vi "Elevator.vi"() -> ()   [LabVIEW 2020]
doc: "Main Vi for the Elevator project that will launch the application and all its submodules"
uses:
  Controller/Controls/Application Event Message.ctl
  Controller/Controls/Application Modules.ctl
  Controller/Controls/Application Events.ctl
  Error Module/Controls/Module Message.ctl
  Configuration Database/Controls/FGV Mode.ctl
  Controller/Controller.lvlib
  Error Module/Error Handler.lvlib
  Configuration Database/Configuration Database.lvlib
  Sensor Interface/Sensor Interface.lvlib
  User Console/User Console.lvlib
  Display Console/Display Console.lvlib
panel:
  in  "Simulate Configuration Database?":bool
  in  "Simulate Sensor Interface?":bool
  in  "Simulate Display Console?":bool
  in  "Simulate User Console?":bool
  out "error out":errorcluster
  in  "error in":errorcluster
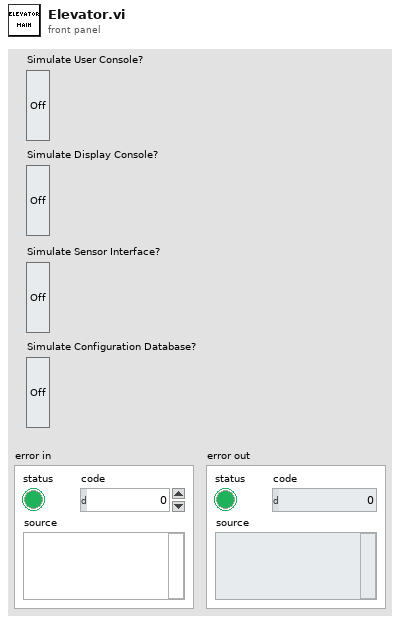
[diagram p1: front panel]
types:
  T1 = typedef "Configuration Database.lvlib/FGV Mode.ctl" = enum16{"Initialize", "Get", "Update", "Close"}
  T2 = typedef "Error Handler.lvlib/Module Message.ctl" = cluster{"Source":T3, "Error":errorcluster}
  T3 = typedef "Controller.lvlib/Application Modules.ctl" = enum16{"Controller", "User Console", "Display Console", "Sensor Interface", "Configuration Database", "Error Module"}
  T4 = typedef "Controller.lvlib/Application Event Message.ctl" = cluster{"Source":T3, "Event":T5, "Data":variant}
  T5 = typedef "Controller.lvlib/Application Events.ctl" = enum16{"Controller: Initialize", "Controller: Initialize Start And Move State", "Controller: Initialize Analysis State", "Controller: Initialize Continue Travel State", "Controller: Initialize Stop At Floor", "Controller: Initialize Open And Close Door Sequence", "Controller: Initialize No Request Remaining", "Controller: Initialize Emergency Call", "Controller: Initialize Terminate Process", "Controller: Publish State", "UI: Elevator Call", "UI: Broadcast State", "UI: Next Destination Reached", "UI: Timeout Reached", "UI: Emergency Call", "UI: Terminate State", "UI: Door Opened", "UI: Door Closed", "UI: Floor Reached", "UI: Door About To Close"}
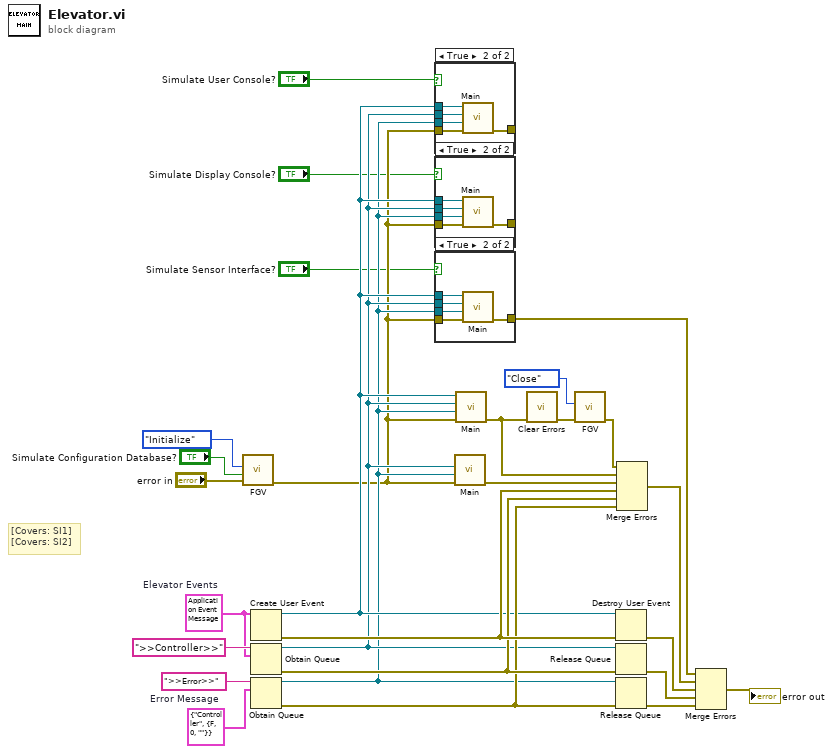
[diagram p0: block diagram]
diagram:
  w21 = T2 {"Source"=enum."Controller", "Error"={"status"=FALSE, "code"=0, "source"=""}}  # Error Message
  w22 = T4 {"Source"=enum."Controller", "Event"=enum."Controller: Initialize", "Data"=variant}  # Elevator Events
  # "[Covers: SI1] \n[Covers: SI2]"
  n1 = call "FGV.vi"("error in"="error in", "Use Simulated?"="Simulate Configuration Database?", "Mode"=FGV_Mode."Initialize") -> ("error out"=w8:errorcluster)  [unwired: 7 in, 1 out]
  n2 = Create User Event(user event datatype=w22) -> (user event=w11:refnum<user-event>, error out=w16:errorcluster)  [unwired: 1 in]
  n3 = Obtain Queue(name (unnamed)=">>Controller>>", element data type=w22) -> (queue out=w10:refnum<queue>, error out=w15:errorcluster)  [unwired: 3 in, 1 out]
  n4 = Obtain Queue(name (unnamed)=">>Error>>", element data type=w21) -> (queue out=w9:refnum<queue>, error out=w14:errorcluster)  [unwired: 3 in, 1 out]
  n5 = case shown="True" "Simulate User Console?" {
    tunnel: w8 -> [w29 w34]
    tunnel: w9 -> [_ w33]
    tunnel: w10 -> [_ w32]
    tunnel: w11 -> [_ w31]
    tunnel: [w29 w30] -> _
    frame False {
    }
    frame True {
      n6 = call "Main.vi"("error in"=w34, "Error Queue"=w33, "Controller Queue"=w32, "Application Events"=w31) -> ("error out"=w30:errorcluster)  [unwired: 7 in]
    }
  }
  n7 = case shown="True" "Simulate Display Console?" {
    tunnel: w8 -> [w35 w40]
    tunnel: w9 -> [_ w39]
    tunnel: w10 -> [_ w38]
    tunnel: w11 -> [_ w37]
    tunnel: [w35 w36] -> _
    frame False {
    }
    frame True {
      n8 = call "Main.vi"("error in"=w40, "Error Queue"=w39, "Controller Queue"=w38, "Application Events"=w37) -> ("error out"=w36:errorcluster)  [unwired: 7 in]
    }
  }
  n9 = case shown="True" "Simulate Sensor Interface?" {
    tunnel: w8 -> [w41 w46]
    tunnel: w9 -> [_ w45]
    tunnel: w10 -> [_ w44]
    tunnel: w11 -> [_ w43]
    tunnel: [w41 w42] -> w12
    frame False {
    }
    frame True {
      n10 = call "Main.vi"("error in"=w46, "Error Queue"=w45, "Controller Queue"=w44, "Application Events"=w43) -> ("error out"=w42:errorcluster)  [unwired: 7 in]
    }
  }
  n11 = call "Main.vi"("error in"=w8, "Error Queue"=w9, "Controller Queue"=w10) -> ("error out"=w17:errorcluster)  [unwired: 8 in]
  n12 = call "Main.vi"("error in"=w8, "Error Queue"=w9, "Controller Queue"=w10, "Application Events"=w11) -> ("error out"=w3:errorcluster)  [unwired: 7 in]
  n13 = call <vilib>:"Clear Errors.vi"("error in (no error)"=w3) -> ("error out"=w2:errorcluster)  [unwired: 5 in, 1 out]
  n14 = call "FGV.vi"("error in"=w2, "Mode"=FGV_Mode."Close") -> ("error out"=w4:errorcluster)  [unwired: 8 in, 1 out]
  n15 = Destroy User Event(user event=w11, error in=w16) -> (error out=w28:errorcluster)
  n16 = Release Queue(queue=w10, error in (no error)=w15) -> (error out=w27:errorcluster)  [unwired: 1 in, 2 out]
  n17 = Release Queue(queue=w9, error in (no error)=w14) -> (error out=w26:errorcluster)  [unwired: 1 in, 2 out]
  n18 = Merge Errors(w4, w3, w17, w16, w15, w14) -> (w13:errorcluster)
  n19 = Merge Errors(w12, w13, w28, w27, w26) -> (→"error out":errorcluster)
